vi "Tanque1.vi"() -> (5 "Numeric":dbl format="%#.2g")   [LabVIEW 2020]
panel:
  in  "Dial":dbl(knob) scale=0.0..100.0
  # "Tanque #1"
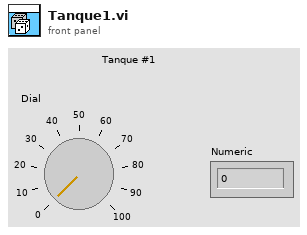
[diagram p1: front panel]
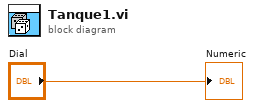
[diagram p0: block diagram]
diagram:
  "Numeric" <- "Dial"
